vi "XL320_ASCII Positions and Times to Dynamixel Positions and Speeds.vi"(8 "Minimum Speed (Max RPM)":u16, 10 "Step Times (ms)":u32[](array[numeric]), 11 "Positions":string[][](array[string])) -> (1 "Dynamixel Speeds":u16[][](array[numeric]), 3 "Dynamixel Positions":u16[][](array[numeric]))   [LabVIEW 2015]
doc: "Accepts a 2D array of positions (2D string) and a corresponding 1D array of step times. The VI calculates the speed needed for each motor to move from one position to the next in the given step time and outputs the Dynamixel speed value with the corresponding Dynamixel position value."
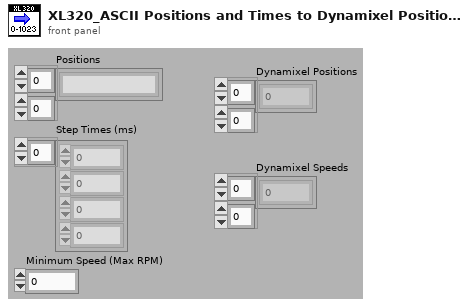
[diagram p1: front panel]
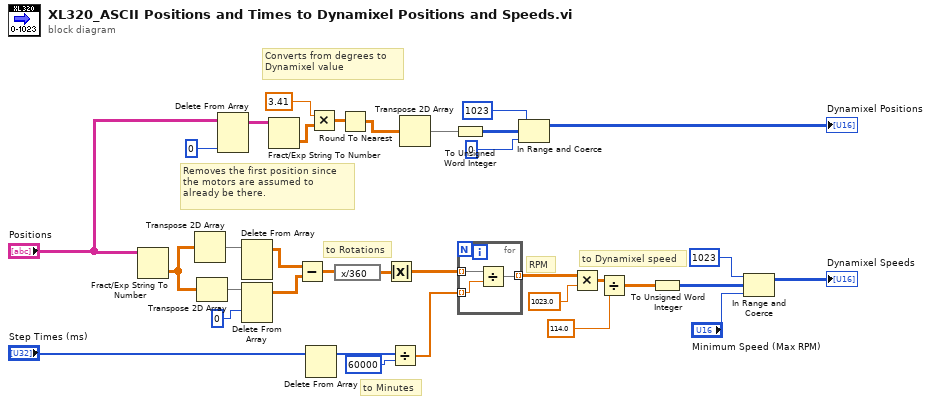
[diagram p0: block diagram]
diagram:
  # "Removes the first position since \nthe motors are assumed to \nalready be there."
  # "Converts from degrees to \nDynamixel value"
  # "to Dynamixel speed"
  # "RPM"
  # "to Minutes"
  # "to Rotations"
  n1 = Fract/Exp String To Number(string="Positions") -> (number=w31:dbl[][])  [unwired: 3 in, 1 out]
  n2 = Transpose 2D Array(2D array=w31) -> (transposed array=w17:dbl[][])
  n3 = Transpose 2D Array(2D array=w31) -> (transposed array=w32:dbl[][])
  n4 = Delete From Array(array="Positions", index (col)=0) -> (array with subset deleted=w27:string[][])  [unwired: 2 in, 1 out]
  n5 = Delete From Array(array=w17) -> (array with subset deleted=w33:dbl[][])  [unwired: 3 in, 1 out]
  n6 = Delete From Array(array=w32, index (row)=0) -> (array with subset deleted=w16:dbl[][])  [unwired: 2 in, 1 out]
  n7 = Fract/Exp String To Number(string=w27) -> (number=w25:dbl[][])  [unwired: 3 in, 1 out]
  n8 = Subtract(x=w33, y=w16) -> (x-y=w21:dbl[][])
  n9 = Delete From Array(array="Step Times (ms)") -> (array with subset deleted=w19:u32[])  [unwired: 2 in, 1 out]
  n10 = Multiply(x=3.41, y=w25) -> (x*y=w24:dbl[][])
  n11 = expression code="x/360"(w21) -> (w22:dbl[][])
  n12 = Round To Nearest(number=w24) -> (nearest integer value=w23:dbl[][])
  n13 = Absolute Value(x=w22) -> (abs(x)=w34:dbl[][])
  n14 = Divide(x=w19, y=60000) -> (x/y=w20:dbl[])
  n15 = Transpose 2D Array(2D array=w23) -> (transposed array=w12:dbl[][])
  n16 = To Unsigned Word Integer(number=w12) -> (unsigned 16bit integer=w10:u16[][])
  n17 = for {
    tunnel: [w37] -> w5 mode=indexing
    tunnel: w34 -> [w36] mode=indexing
    tunnel: w20 -> [w35] mode=indexing
    n18 = Divide(x=w36, y=w35) -> (x/y=w37:dbl[])
  }
  n19 = In Range and Coerce(upper limit=u16 1023, x=w10, lower limit=u16 0) -> (coerced(x)=→"Dynamixel Positions":u16[][])  [unwired: 1 out]
  n20 = Multiply(x=w5, y=1023.0) -> (x*y=w6:dbl[][])
  n21 = Divide(x=w6, y=114.0) -> (x/y=w3:dbl[][])
  n22 = To Unsigned Word Integer(number=w3) -> (unsigned 16bit integer=w2:u16[][])
  n23 = In Range and Coerce(upper limit=u16 1023, x=w2, lower limit="Minimum Speed (Max RPM)") -> (coerced(x)=→"Dynamixel Speeds":u16[][])  [unwired: 1 out]
